vi "StepDigVoltage.vi"(2 "Digitizer Settings":T1={"Digitizer delay (us) "=0.0, "rf points per line"=2048, "lines per plane"=128, "Samp Rate (Hz)"=100000000.0, "Additional dig delay (us)"=0.0, "Voltage Scale"=0.4, "Pre-Looks"=0, "Offset delay (us)"=0.0, "bits A/D"=8, "Avg Num"=1, "DigTimeOut"=5.0, "Rel Dig Delay"=0.0, "Dig Ch"=0, "LeCroyCluster"={"LeCroy Channels"=[TRUE, FALSE, FALSE, FALSE], "LC read pt offset"=0.0, "Sweep Avg"=FALSE}, "Main Digitizer"=enum."NI Digitizer", "Dig Config"=enum."Single channel", "Digitizer ID Cluster"={"Acqiris/Alazar/SP ID"=[], "NI Instr Handles"=[], "LeCroy VISA"="", "GaGe Handle"={"Handle"=0, "Sample size"=0, "Resolution"=0, "Offset"=0, "Channels"=0, "Boards"=0}, "ATS Ref"="ATS9350", "Acqiris Address"=["PCI::INSTR0"], "ADQRef"=refnum, "adq_cu_ptr"=refnum}, "Trigger Settings"={"Trig Source"=1, "Trig Coupling"=0, "Trig Slope"=0, "Level (mV)"=1500.0}, "Bulk Acq"=FALSE, "Bulk Start Indexes"=[], "Data Ref RF"=refnum, "NI ID/Channel"=[], "Total Dig CH"=1, "Xtra Ann Trig delay (us)"=10.0, "Fix Z Delay?"=FALSE, "One Way Transmission?"=FALSE, "Data Ref Log"=refnum} {"Trigger Settings"."Trig Slope" items=["Positive", "Negative"]; "Trigger Settings"."Level (mV)" format="%.2f"; "Trigger Settings"."Trig Coupling" items=["DC 1 MOhm", "AC 1 MOhm", "DC 50 Ohm", "AC 50 Ohm"]; "Trigger Settings"."Trig Source" items=["Chan 1", "External"]; "Rel Dig Delay" format="%.2f"; "DigTimeOut" format="%.2f"; "Avg Num" min=1; "Offset delay (us)" format="%.2f"; "Additional dig delay (us)" format="%.2f"; "Digitizer delay (us)" format="%.2f"}, 3 "Voltage Settings":T5, 4 "Prev Vol Val":i16) -> ()   [LabVIEW 2022 SP3]
uses:
  DigitizerSettings.ctl
  Digitizer.ctl
  DigConfig.ctl
  DigitizerID.ctl
  C:/Windows/System32/ADQAPI_dotNet_helper.dll
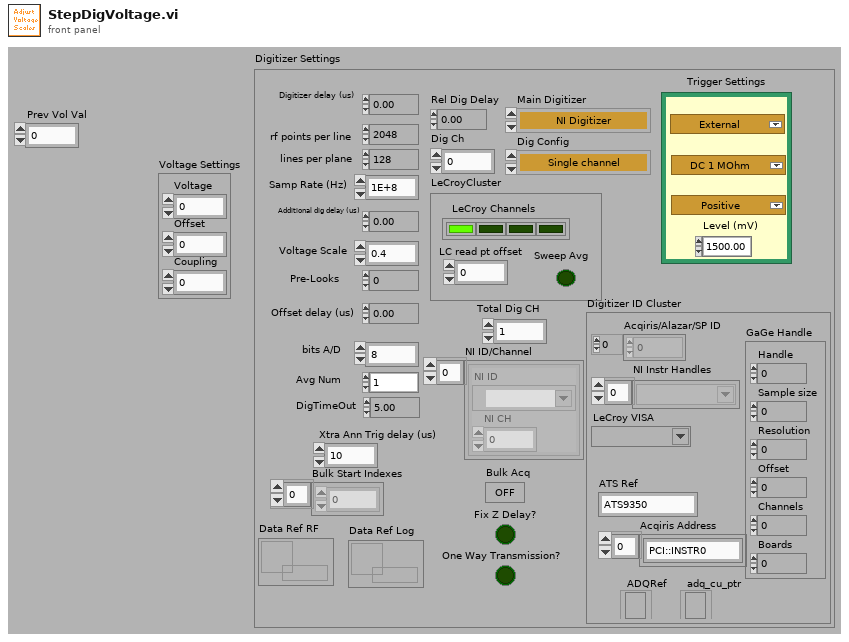
[diagram p1: front panel]
types:
  T1 = typedef "DigitizerSettings.ctl" = cluster{"Digitizer delay (us) ":dbl, "rf points per line":i32, "lines per plane":i32, "Samp Rate (Hz)":dbl, "Additional dig delay (us)":dbl, "Voltage Scale":dbl, "Pre-Looks":i32, "Offset delay (us)":dbl, "bits A/D":i8, "Avg Num":i32, "DigTimeOut":sgl, "Rel Dig Delay":sgl, "Dig Ch":i32, "LeCroyCluster":cluster{"LeCroy Channels":bool[], "LC read pt offset":dbl, "Sweep Avg":bool}, "Main Digitizer":T2, "Dig Config":T3, "Digitizer ID Cluster":T4, "Trigger Settings":cluster{"Trig Source":u16, "Trig Coupling":u16, "Trig Slope":u16, "Level (mV)":dbl}, "Bulk Acq":bool, "Bulk Start Indexes":i32[], "Data Ref RF":refnum<data-value>, "NI ID/Channel":cluster{"NI ID":refnum<k15>, "NI CH":i32}[], "Total Dig CH":i32, "Xtra Ann Trig delay (us)":dbl, "Fix Z Delay?":bool, "One Way Transmission?":bool, "Data Ref Log":refnum<data-value>}
  T2 = typedef "Digitizer.ctl" = enum16{"Acqiris Digitizer", "NI Digitizer", "LeCroy", "GaGe", "AlazarTech", "No Digitizer", "Teledyne"}
  T3 = typedef "DigConfig.ctl" = enum16{"Single channel", "2 Chans w/ 2 Acqiris", "2 Chans w/ 1 Acqiris", "5-CH Pulser New", "5-CH pulser w/ ann array", "5-pass style ann array", "Empty"}
  T4 = typedef "DigitizerID.ctl" = cluster{"Acqiris/Alazar/SP ID":u32[], "NI Instr Handles":refnum<k15>[], "LeCroy VISA":refnum<visa-resource-name>, "GaGe Handle":cluster{"Handle":u32, "Sample size":u32, "Resolution":i32, "Offset":i32, "Channels":u32, "Boards":u32}, "ATS Ref":string, "Acqiris Address":string[], "ADQRef":refnum<k24>, "adq_cu_ptr":refnum<k24>}
  T5 = cluster{"Voltage":dbl, "Offset":dbl, "Coupling":u16}
  T6 = cluster{"Voltage Scale":i16, "Offset":dbl, "Coupling":u16}
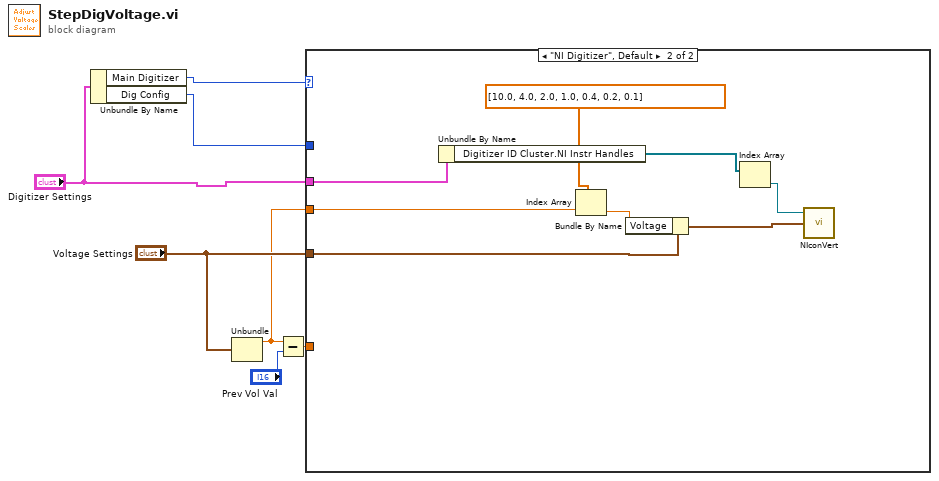
[diagram p0: block diagram]
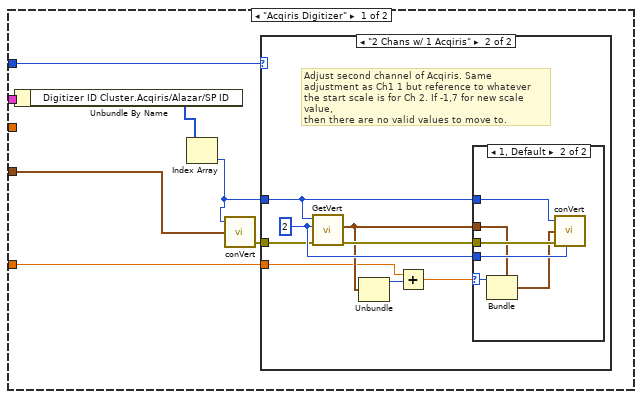
[diagram p2: hidden frame]
diagram:
  n1 = Unbundle By Name("Digitizer Settings") -> ("Main Digitizer"=w2:T2, "Dig Config"=w1:T3)
  n2 = Unbundle("Voltage Settings") -> ("Voltage"=w4:dbl)  [unwired: 2 out]
  n3 = Subtract(x=w4, y="Prev Vol Val") -> (x-y=w5:dbl)
  n4 = case shown="\"NI Digitizer\", Default" w2 {
    tunnel: "Voltage Settings" -> [w13 w35]
    tunnel: w1 -> [w14 _]
    tunnel: w5 -> [w11 _]
    tunnel: w4 -> [_ w33]
    tunnel: "Digitizer Settings" -> [w10 w30]
    frame "Acqiris Digitizer" {
      n5 = Unbundle By Name(w10) -> ("Digitizer ID Cluster.Acqiris/Alazar/SP ID"=w9:u32[])
      n6 = Index Array(array=w9) -> (element=w8:u32)  [unwired: 1 in]
      n7 = call "conVert.vi"("InstrumentID"=w8, "V scale"=w13) -> ("error out"=w12:errorcluster)  [unwired: 2 in, 3 out]
      n8 = case shown="\"2 Chans w/ 1 Acqiris\"" w14 {
        tunnel: w8 -> [_ w22]
        tunnel: w12 -> [_ w20]
        tunnel: w11 -> [_ w17]
        frame "Single channel", Default {
        }
        frame "2 Chans w/ 1 Acqiris" {
          w21 = 2 ("Channel (1)")
          # "Adjust second channel of Acqiris. Same adjustment as Ch1 1 but reference to whatever the start scale is for Ch 2. If -1,7 for new scale value,\nthen there are no valid values to move to."
          n9 = call "GetVert.vi"("error in"=w20, "Channel (1)"=w21, "InstrumentID"=w22) -> ("error out"=w19:errorcluster, "V scale"=w18:T6)  [unwired: 1 in, 2 out]
          n10 = Unbundle(w18) -> ("Voltage Scale"=w16:i16)  [unwired: 2 out]
          n11 = Add(x=w17, y=w16) -> (x+y=w15:dbl)
          n12 = case shown="1, Default" w15 {
            selector: w15 -> [_ w23]
            tunnel: w22 -> [_ w28]
            tunnel: w21 -> [_ w27]
            tunnel: w19 -> [_ w26]
            tunnel: w18 -> [_ w25]
            frame -1, 7 {
            }
            frame 1, Default {
              n13 = Bundle(cluster=w25, "Voltage Scale"=w23) -> (w24:T6)  [unwired: 2 in]
              n14 = call "conVert.vi"("InstrumentID"=w28, "V scale"=w24, "error in"=w26, "Channel (1)"=w27) -> ()  [unwired: 4 out]
            }
          }
        }
      }
    }
    frame "NI Digitizer", Default {
      n15 = Unbundle By Name(w30) -> ("Digitizer ID Cluster.NI Instr Handles"=w29:refnum<k15>[])
      n16 = Index Array(array=dbl[] [10.0, 4.0, 2.0, 1.0, 0.4, 0.2, 0.1], index=w33) -> (element=w32:dbl)
      n17 = Bundle By Name(cluster=w35, "Voltage"=w32) -> (w31:T5)
      n18 = Index Array(array=w29) -> (element=w36:refnum<k15>)  [unwired: 1 in]
      n19 = call "NIconVert.vi"("InstrumentID"=w36, "V scale"=w31) -> ()  [unwired: 2 in, 4 out]
    }
  }
